vi "Ask for Connected Device.vi"(7 "GenericDevice.lvclass":refnum<class "GenericDevice.lvclass">, 8 "error in (no error)":errorcluster, 10 "Delay between send and receive [ms]":u32, 11 "Communicator in":refnum<class "Communicator.lvclass">) -> (0 "error out":errorcluster)   [LabVIEW 2023, in "DeviceManager.lvlib"]
uses:
  DeviceManager.lvlib
  Classes/Communicator/Communicator.lvclass
  Classes/GenericDevice/GenericDevice.lvclass
panel:
  out "Communicator out":refnum<class "Communicator.lvclass">
  out "Data":string
  # "Connector Pane"
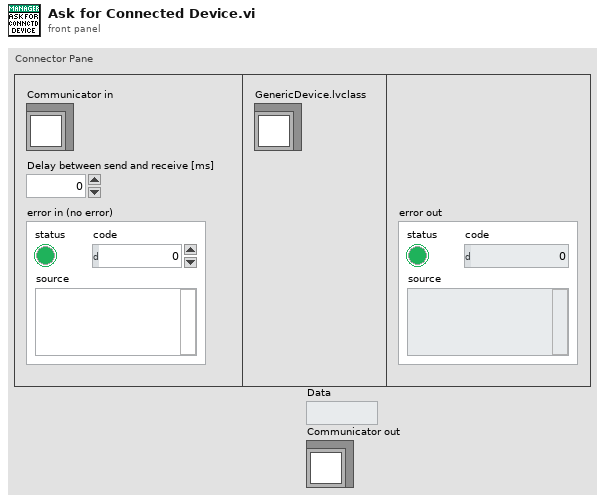
[diagram p1: front panel]
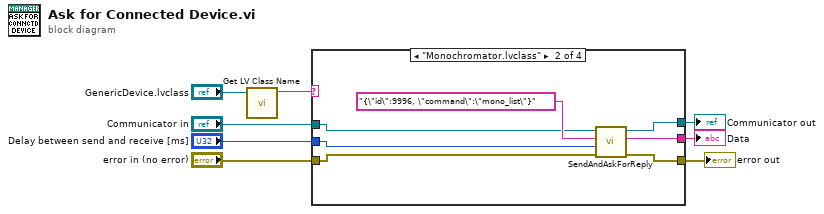
[diagram p0: block diagram]
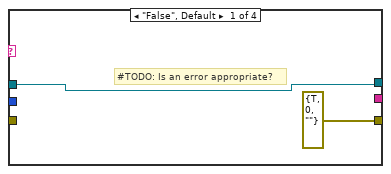
[diagram p2: hidden frame]
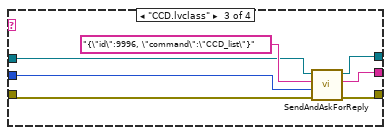
[diagram p3: hidden frame]
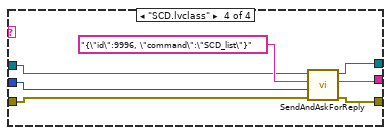
[diagram p4: hidden frame]
diagram:
  n1 = call <vilib>:"Get LV Class Name.vi"("object"="GenericDevice.lvclass") -> ("class name"=w7:string)  [unwired: 9 in, 1 out]
  n2 = case shown="\"Monochromator.lvclass\"" w7 {
    tunnel: "Communicator in" -> [w9 w16 w23 w30]
    tunnel: "Delay between send and receive [ms]" -> [_ w15 w20 w29]
    tunnel: "error in (no error)" -> [_ w14 w21 w28]
    tunnel: [errorcluster {"status"=TRUE, "code"=0, "source"=""} ("error in (no error)") w13 w22 w27] -> w3
    tunnel: [_ w12 w19 w26] -> w2
    tunnel: [w9 w11 w18 w25] -> w1
    frame "False", Default {
      # "#TODO: Is an error appropriate?"
    }
    frame "Monochromator.lvclass" {
      n3 = call-dynamic "SendAndAskForReply.vi"("error in (no error)"=w14, "timeout for receiving data [ms]"=w15, "String to be sent"="{\"id\":9996, \"command\":\"mono_list\"}", "Communicator in"=w16) -> ("error out"=w13:errorcluster, "Data"=w12:string, "Communicator out"=w11:refnum<class "Communicator.lvclass">)  [unwired: 5 in]
    }
    frame "CCD.lvclass" {
      n4 = call-dynamic "SendAndAskForReply.vi"("error in (no error)"=w21, "timeout for receiving data [ms]"=w20, "String to be sent"="{\"id\":9996, \"command\":\"CCD_list\"}", "Communicator in"=w23) -> ("error out"=w22:errorcluster, "Data"=w19:string, "Communicator out"=w18:refnum<class "Communicator.lvclass">)  [unwired: 5 in]
    }
    frame "SCD.lvclass" {
      n5 = call-dynamic "SendAndAskForReply.vi"("error in (no error)"=w28, "timeout for receiving data [ms]"=w29, "String to be sent"="{\"id\":9996, \"command\":\"SCD_list\"}", "Communicator in"=w30) -> ("error out"=w27:errorcluster, "Data"=w26:string, "Communicator out"=w25:refnum<class "Communicator.lvclass">)  [unwired: 5 in]
    }
  }
  "error out" <- w3
  "Data" <- w2
  "Communicator out" <- w1
